vi "Move to Position from File.vi"(8 "error in (no error)":errorcluster, 9 "file path in":path, 11 "VISA in":refnum<visa-resource-name>) -> (0 "error out":errorcluster, 1 "file path out":path, 3 "VISA out":refnum<visa-resource-name>)   [LabVIEW 2018, in "ASI TG-1000.lvlib"]
doc: "Queries the ASI controller for the position along the specified axes and saves the result to a file for later use."
uses:
  ASI TG-1000.lvlib
  Utility/Axis Name.ctl
  Private/File action if doesn't exist.ctl
  <vilib>/Utility/config.llb/Read Key (Double).vi
  <vilib>/Utility/config.llb/NI_LVConfig.lvlib
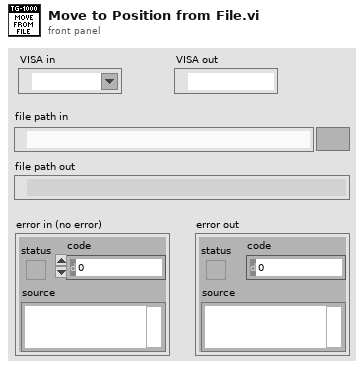
[diagram p1: front panel]
types:
  T1 = typedef "ASI TG-1000.lvlib/File action if doesn't exist.ctl" = enum16{"prompt for existing", "try to create, prompt if can't", "try to create, error if can't"}
  T2 = typedef "ASI TG-1000.lvlib/Axis Name.ctl" = enum8{"undefined", "A", "B", "C", "D", "E", "F", "G", "H", "I", "J", "K", "L", "M", "N", "O", "P", "Q", "R", "S", "T", "U", "V", "W", "X", "Y", "Z"}
  T3 = typedef "NI_LVConfig.lvlib/Config Data RefNum.ctl" = refnum<k1>
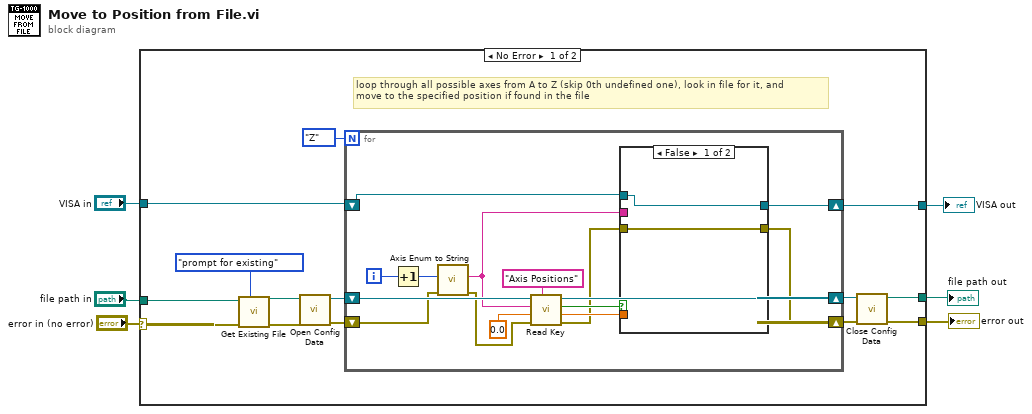
[diagram p0: block diagram]
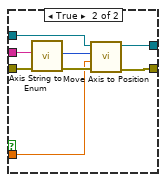
[diagram p2: hidden frame]
diagram:
  n1 = case shown="No Error" "error in (no error)" {
    selector: "error in (no error)" -> [w12 w48]
    tunnel: [w20 w48] -> w6
    tunnel: "VISA in" -> [w19 w47]
    tunnel: [w18 w47] -> w3
    tunnel: [w8 w46] -> w2
    tunnel: "file path in" -> [w7 w46]
    frame No Error {
      # "loop through all possible axes from A to Z (skip 0th undefined one), look in file for it, and \nmove to the specified position if found in the file"
      n2 = call "Get Existing File.vi"("action if file doesn't exist (0: prompt for existing)"=File_action_if_doesn't_exist."prompt for existing" ("action if doesn't exist (0: prompt for existing)"), "error in (no error)"=w12, "file path in"=w7) -> ("error out"=w11:errorcluster, "file path out"=w10:path)  [unwired: 7 in]
      n3 = call <vilib>:"Open Config Data.vi"("error in (no error)"=w11, "configuration file path"=w10) -> ("error out"=w16:errorcluster, "refnum"=w17:T3)  [unwired: 7 in, 1 out]
      n4 = for {
        N: Axis_Name."Z" ("Axis") -> [_]
        shift-right: [w33] -> w15
        shift-left: w17 -> [w35]
        shift-right: [w23] -> w14
        shift-left: w16 -> [w22]
        shift-right: [w26] -> w18
        shift-left: w19 -> [w25]
        i -> [w31]
        n5 = Increment(x=w31) -> (x+1=w24:i32)
        n6 = call "Axis Enum to String.vi"("error in (no error)"=w22, "Axis Enum In"=w24) -> ("error out"=w21:errorcluster, "Axis String Out"=w29:string)  [unwired: 8 in]
        n7 = call-poly <vilib>:"Read Key.vi"("section"="Axis Positions", "error in (no error)"=w21, "default value"=0.0, "key"=w29, "refnum"=w35) -> ("error out"=w27:errorcluster, "value"=w28:dbl, "found?"=w30:bool, "refnum out"=w33:T3)  [unwired: 3 in]
        n8 = case shown="False" w30 {
          tunnel: w29 -> [_ w45]
          tunnel: w28 -> [_ w38]
          tunnel: w27 -> [w36 w44]
          tunnel: [w36 w42] -> w23
          tunnel: [w37 w41] -> w26
          tunnel: w25 -> [w37 w40]
          frame False {
          }
          frame True {
            n9 = call "Axis String to Enum.vi"("error in (no error)"=w44, "Axis String In"=w45) -> ("error out"=w43:errorcluster, "Axis Enum Out"=w39:T2)  [unwired: 8 in]
            n10 = call "Move Axis to Position.vi"("error in (no error)"=w43, "Position [internal units]"=w38, "Axis"=w39, "VISA in"=w40) -> ("error out"=w42:errorcluster, "VISA out"=w41:refnum<visa-resource-name>)  [unwired: 5 in]
          }
        }
      }
      n11 = call <vilib>:"Close Config Data.vi"("error in (no error)"=w14, "refnum"=w15) -> ("error out"=w20:errorcluster, "file path"=w8:path)  [unwired: 8 in]
    }
    frame Error {
    }
  }
  "error out" <- w6
  "VISA out" <- w3
  "file path out" <- w2
